vi "canDataSort.vi"() -> ()   [LabVIEW 2023] (continued)
  0CF103A7   00000004    8        17\t1F\t08\t60\tB1\t1F\t08\t66\r\n      4644  0C3C4D4A   00000004    8        BE\tFF\tFF\t7F\t18\tFF\tFF\t66\r\n      4643  0CF102A7   00000004    8        30\t75\tE0\t2E\t80\tFF\tFF\tFD\r\n      4642  0CF101A7   00000004    8        68\t00\t97\tCC\t00\t19\t39\t02\r\n      4649  18FEF117   00000004    8        F7\t97\tCC\tCF\tFF\tFF\tFF\tFF\r\n      4648  18FB01A7   00000004    8        FF\t1F\tFF\tFF\tFF\tFF\tFF\tFF\r\n      4648  18F121F0   00000004    8        09\t34\t00\t00\tFF\tFF\tB0\t01\r\n      4647  18F120F0   00000004    8        2B\t75\t60\tB1\tB0\t01\tFF\tFF\r\n      4646  18F108A7   00000004    8        F0\t00\t00\tFF\tFF\tFF\tFF\t47\r\n      4646  18F106A7   00000004    8        00\tF7\tFF\tFF\tFF\tFF\tFF\tCD\r\n      4645  0CF105A7   00000004    8        94\t11\t00\t55\tFF\tFF\tFF\t23\r\n      4645  0CF104A7   00000004    8        F0\t60\t22\tFC\tFF\tFF\tFF\t66\r\n      4644  0CF103A7   00000004    8        17\t1F\t08\t60\tB1\t1F\t08\t66\r\n      4644  0C3C4D4A   00000004    8        BE\tFF\tFF\t7F\t18\tFF\tFF\t66\r\n      4643  0CF102A7   00000004    8        30\t75\tE0\t2E\t80\tFF\tFF\tFD\r\n      4649  1FFFFFFF   00000004    8        00\t00\tFF\tFF\tFF\tFF\tFF\tFF\r\n      4649  18FEF117   00000004    8        F7\t97\tCC\tCF\tFF\tFF\tFF\tFF\r\n      4648  18FB01A7   00000004    8        FF\t1F\tFF\tFF\tFF\tFF\tFF\tFF\r\n      4648  18F121F0   00000004    8        09\t34\t00\t00\tFF\tFF\tB0\t01\r\n      4647  18F120F0   00000004    8        2B\t75\t60\tB1\tB0\t01\tFF\tFF\r\n      4646  18F108A7   00000004    8        F0\t00\t00\tFF\tFF\tFF\tFF\t47\r\n      4646  18F106A7   00000004    8        00\tF7\tFF\tFF\tFF\tFF\tFF\tCD\r\n      4645  0CF105A7   00000004    8        94\t11\t00\t55\tFF\tFF\tFF\t23\r\n      4645  0CF104A7   00000004    8        F0\t60\t22\tFC\tFF\tFF\tFF\t66\r\n      4644  0CF103A7   00000004    8        17\t1F\t08\t60\tB1\t1F\t08\t66\r\n      4644  0C3C4D4A   00000004    8        BE\tFF\tFF\t7F\t18\tFF\tFF\t66\r\n      4652  1FFFFFFF   00000004    8        00\t20\tFF\tFF\tFF\tFF\tFF\tFF\r\n      4649  1FFFFFFF   00000004    8        00\t00\tFF\tFF\tFF\tFF\tFF\tFF\r\n      4649  18FEF117   00000004    8        F7\t97\tCC\tCF\tFF\tFF\tFF\tFF\r\n      4648  18FB01A7   00000004    8        FF\t1F\tFF\tFF\tFF\tFF\tFF\tFF\r\n      4648  18F121F0   00000004    8        09\t34\t00\t00\tFF\tFF\tB0\t01\r\n      4647  18F120F0   00000004    8        2B\t75\t60\tB1\tB0\t01\tFF\tFF\r\n      4646  18F108A7   00000004    8        F0\t00\t00\tFF\tFF\tFF\tFF\t47\r\n      4646  18F106A7   00000004    8        00\tF7\tFF\tFF\tFF\tFF\tFF\tCD\r\n      4645  0CF105A7   00000004    8        94\t11\t00\t55\tFF\tFF\tFF\t23\r\n      4645  0CF104A7   00000004    8        F0\t60\t22\tFC\tFF\tFF\tFF\t66\r\n      4644  0CF103A7   00000004    8        17\t1F\t08\t60\tB1\t1F\t08\t66\r\n      4662  1FFFFFFF   00000004    8        00\t20\tFF\tFF\tFF\tFF\tFF\tFF\r\n      4652  1FFFFFFF   00000004    8        00\t20\tFF\tFF\tFF\tFF\tFF\tFF\r\n      4649  1FFFFFFF   00000004    8        00\t00\tFF\tFF\tFF\tFF\tFF\tFF\r\n      4649  18FEF117   00000004    8        F7\t97\tCC\tCF\tFF\tFF\tFF\tFF\r\n      4648  18FB01A7   00000004    8        FF\t1F\tFF\tFF\tFF\tFF\tFF\tFF\r\n      4648  18F121F0   00000004    8        09\t34\t00\t00\tFF\tFF\tB0\t01\r\n      4647  18F120F0   00000004    8        2B\t75\t60\tB1\tB0\t01\tFF\tFF\r\n      4646  18F108A7   00000004    8        F0\t00\t00\tFF\tFF\tFF\tFF\t47\r\n      4646  18F106A7   00000004    8        00\tF7\tFF\tFF\tFF\tFF\tFF\tCD\r\n      4645  0CF105A7   00000004    8        94\t11\t00\t55\tFF\tFF\tFF\t23\r\n      4645  0CF104A7   00000004    8        F0\t60\t22\tFC\tFF\tFF\tFF\t66\r\n      4662  0CF101A7   00000004    8        68\t00\t97\tCC\t00\t19\t39\t03\r\n      4662  1FFFFFFF   00000004    8        00\t20\tFF\tFF\tFF\tFF\tFF\tFF\r\n      4652  1FFFFFFF   00000004    8        00\t20\tFF\tFF\tFF\tFF\tFF\tFF\r\n      4649  1FFFFFFF   00000004    8        00\t00\tFF\tFF\tFF\tFF\tFF\tFF\r\n      4649  18FEF117   00000004    8        F7\t97\tCC\tCF\tFF\tFF\tFF\tFF\r\n      4648  18FB01A7   00000004    8        FF\t1F\tFF\tFF\tFF\tFF\tFF\tFF\r\n      4648  18F121F0   00000004    8        09\t34\t00\t00\tFF\tFF\tB0\t01\r\n      4647  18F120F0   00000004    8        2B\t75\t60\tB1\tB0\t01\tFF\tFF\r\n      4646  18F108A7   00000004    8        F0\t00\t00\tFF\tFF\tFF\tFF\t47\r\n      4646  18F106A7   00000004    8        00\tF7\tFF\tFF\tFF\tFF\tFF\tCD\r\n      4645  0CF105A7   00000004    8        94\t11\t00\t55\tFF\tFF\tFF\t23\r\n      4663  0CF102A7   00000004    8        30\t75\tE0\t2E\t80\tFF\tFF\tFD\r\n      4662  0CF101A7   00000004    8        68\t00\t97\tCC\t00\t19\t39\t03\r\n      4662  1FFFFFFF   00000004    8        00\t20\tFF\tFF\tFF\tFF\tFF\tFF\r\n      4652  1FFFFFFF   00000004    8        00\t20\tFF\tFF\tFF\tFF\tFF\tFF\r\n      4649  1FFFFFFF   00000004    8        00\t00\tFF\tFF\tFF\tFF\tFF\tFF\r\n      4649  18FEF117   00000004    8        F7\t97\tCC\tCF\tFF\tFF\tFF\tFF\r\n      4648  18FB01A7   00000004    8        FF\t1F\tFF\tFF\tFF\tFF\tFF\tFF\r\n      4648  18F121F0   00000004    8        09\t34\t00\t00\tFF\tFF\tB0\t01\r\n      4647  18F120F0   00000004    8        2B\t75\t60\tB1\tB0\t01\tFF\tFF\r\n      4646  18F108A7   00000004    8        F0\t00\t00\tFF\tFF\tFF\tFF\t47\r\n      4646  18F106A7   00000004    8        00\tF7\tFF\tFF\tFF\tFF\tFF\tCD\r\n      4672  1FFFFFFF   00000004    8        00\t20\tFF\tFF\tFF\tFF\tFF\tFF\r\n      4663  0CF102A7   00000004    8        30\t75\tE0\t2E\t80\tFF\tFF\tFD\r\n      4662  0CF101A7   00000004    8        68\t00\t97\tCC\t00\t19\t39\t03\r\n      4662  1FFFFFFF   00000004    8        00\t20\tFF\tFF\tFF\tFF\tFF\tFF\r\n      4652  1FFFFFFF   00000004    8        00\t20\tFF\tFF\tFF\tFF\tFF\tFF\r\n      4649  1FFFFFFF   00000004    8        00\t00\tFF\tFF\tFF\tFF\tFF\tFF\r\n      4649  18FEF117   00000004    8        F7\t97\tCC\tCF\tFF\tFF\tFF\tFF\r\n      4648  18FB01A7   00000004    8        FF\t1F\tFF\tFF\tFF\tFF\tFF\tFF\r\n      4648  18F121F0   00000004    8        09\t34\t00\t00\tFF\tFF\tB0\t01\r\n      4647  18F120F0   00000004    8        2B\t75\t60\tB1\tB0\t01\tFF\tFF\r\n      4646  18F108A7   00000004    8        F0\t00\t00\tFF\tFF\tFF\tFF\t47\r\n      4682  1FFFFFFF   00000004    8        00\t20\tFF\tFF\tFF\tFF\tFF\tFF\r\n      4672  1FFFFFFF   00000004    8        00\t20\tFF\tFF\tFF\tFF\tFF\tFF\r\n      4663  0CF102A7   00000004    8        30\t75\tE0\t2E\t80\tFF\tFF\tFD\r\n      4662  0CF101A7   00000004    8        68\t00\t97\tCC\t00\t19\t39\t03\r\n      4662  1FFFFFFF   00000004    8        00\t20\tFF\tFF\tFF\tFF\tFF\tFF\r\n      4652  1FFFFFFF   00000004    8        00\t20\tFF\tFF\tFF\tFF\tFF\tFF\r\n      4649  1FFFFFFF   00000004    8        00\t00\tFF\tFF\tFF\tFF\tFF\tFF\r\n      4649  18FEF117   00000004    8        F7\t97\tCC\tCF\tFF\tFF\tFF\tFF\r\n      4648  18FB01A7   00000004    8        FF\t1F\tFF\tFF\tFF\tFF\tFF\tFF\r\n      4648  18F121F0   00000004    8        09\t34\t00\t00\tFF\tFF\tB0\t01\r\n      4647  18F120F0   00000004    8        2B\t75\t60\tB1\tB0\t01\tFF\tFF\r\n      4683  0CF101A7   00000004    8        68\t00\t97\tCC\t00\t19\t39\t04\r\n      4682  1FFFFFFF   00000004    8        00\t20\tFF\tFF\tFF\tFF\tFF\tFF\r\n      4672  1FFFFFFF   00000004    8        00\t20\tFF\tFF\tFF\tFF\tFF\tFF\r\n      4663  0CF102A7   00000004    8        30\t75\tE0\t2E\t80\tFF\tFF\tFD\r\n      4662  0CF101A7   00000004    8        68\t00\t97\tCC\t00\t19\t39\t03\r\n      4662  1FFFFFFF   00000004    8        00\t20\tFF\tFF\tFF\tFF\tFF\tFF\r\n      4652  1FFFFFFF   00000004    8        00\t20\tFF\tFF\tFF\tFF\tFF\tFF\r\n      4649  1FFFFFFF   00000004    8        00\t00\tFF\tFF\tFF\tFF\tFF\tFF\r\n      4649  18FEF117   00000004    8        F7\t97\tCC\tCF\tFF\tFF\tFF\tFF\r\n      4648  18FB01A7   00000004    8        FF\t1F\tFF\tFF\tFF\tFF\tFF\tFF\r\n      4648  18F121F0   00000004    8        09\t34\t00\t00\tFF\tFF\tB0\t01\r\n      4683  0CF102A7   00000004    8        30\t75\tE0\t2E\t80\tFF\tFF\tFD\r\n      4683  0CF101A7   00000004    8        68\t00\t97\tCC\t00\t19\t39\t04\r\n      4682  1FFFFFFF   00000004    8        00\t20\tFF\tFF\tFF\tFF\tFF\tFF\r\n      4672  1FFFFFFF   00000004    8        00\t20\tFF\tFF\tFF\tFF\tFF\tFF\r\n      4663  0CF102A7   00000004    8        30\t75\tE0\t2E\t80\tFF\tFF\tFD\r\n      4662  0CF101A7   00000004    8        68\t00\t97\tCC\t00\t19\t39\t03\r\n      4662  1FFFFFFF   00000004    8        00\t20\tFF\tFF\tFF\tFF\tFF\tFF\r\n      4652  1FFFFFFF   00000004    8        00\t20\tFF\tFF\tFF\tFF\tFF\tFF\r\n      4649  1FFFFFFF   00000004    8        00\t00\tFF\tFF\tFF\tFF\tFF\tFF\r\n      4649  18FEF117   00000004    8        F7\t97\tCC\tCF\tFF\tFF\tFF\tFF\r\n      4648  18FB01A7   00000004    8        FF\t1F\tFF\tFF\tFF\tFF\tFF\tFF\r\n      4692  1FFFFFFF   00000004    8        00\t00\tFF\tFF\tFF\tFF\tFF\tFF\r\n      4683  0CF102A7   00000004    8        30\t75\tE0\t2E\t80\tFF\tFF\tFD\r\n      4683  0CF101A7   00000004    8        68\t00\t97\tCC\t00\t19\t39\t04\r\n      4682  1FFFFFFF   00000004    8        00\t20\tFF\tFF\tFF\tFF\tFF\tFF\r\n      4672  1FFFFFFF   00000004    8        00\t20\tFF\tFF\tFF\tFF\tFF\tFF\r\n      4663  0CF102A7   00000004    8        30\t75\tE0\t2E\t80\tFF\tFF\tFD\r\n      4662  0CF101A7   00000004    8        68\t00\t97\tCC\t00\t19\t39\t03\r\n      4662  1FFFFFFF   00000004    8        00\t20\tFF\tFF\tFF\tFF\tFF\tFF\r\n      4652  1FFFFFFF   00000004    8        00\t20\tFF\tFF\tFF\tFF\tFF\tFF\r\n      4649  1FFFFFFF   00000004    8        00\t00\tFF\tFF\tFF\tFF\tFF\tFF\r\n      4649  18FEF117   00000004    8        F7\t97\tCC\tCF\tFF\tFF\tFF\tFF\r\n      4693  18F106A7   00000004    8        00\tF7\tFF\tFF\tFF\tFF\tFF\tCE\r\n      4692  1FFFFFFF   00000004    8        00\t00\tFF\tFF\tFF\tFF\tFF\tFF\r\n      4683  0CF102A7   00000004    8        30\t75\tE0\t2E\t80\tFF\tFF\tFD\r\n      4683  0CF101A7   00000004    8        68\t00\t97\tCC\t00\t19\t39\t04\r\n      4682  1FFFFFFF   00000004    8        00\t20\tFF\tFF\tFF\tFF\tFF\tFF\r\n      4672  1FFFFFFF   00000004    8        00\t20\tFF\tFF\tFF\tFF\tFF\tFF\r\n      4663  0CF102A7   00000004    8        30\t75\tE0\t2E\t80\tFF\tFF\tFD\r\n      4662  0CF101A7   00000004    8        68\t00\t97\tCC\t00\t19\t39\t03\r\n      4662  1FFFFFFF   00000004    8        00\t20\tFF\tFF\tFF\tFF\tFF\tFF\r\n      4652  1FFFFFFF   00000004    8        00\t20\tFF\tFF\tFF\tFF\tFF\tFF\r\n      4649  1FFFFFFF   00000004    8        00\t00\tFF\tFF\tFF\tFF\tFF\tFF\r\n      4702  1FFFFFFF   00000004    8        00\t20\tFF\tFF\tFF\tFF\tFF\tFF\r\n      4693  18F106A7   00000004    8        00\tF7\tFF\tFF\tFF\tFF\tFF\tCE\r\n      4692  1FFFFFFF   00000004    8        00\t00\tFF\tFF\tFF\tFF\tFF\tFF\r\n      4683  0CF102A7   00000004    8        30\t75\tE0\t2E\t80\tFF\tFF\tFD\r\n      4683  0CF101A7   00000004    8        68\t00\t97\tCC\t00\t19\t39\t04\r\n      4682  1FFFFFFF   00000004    8        00\t20\tFF\tFF\tFF\tFF\tFF\tFF\r\n      4672  1FFFFFFF   00000004    8        00\t20\tFF\tFF\tFF\tFF\tFF\tFF\r\n      4663  0CF102A7   00000004    8        30\t75\tE0\t2E\t80\tFF\tFF\tFD\r\n      4662  0CF101A7   00000004    8        68\t00\t97\tCC\t00\t19\t39\t03\r\n      4662  1FFFFFFF   00000004    8        00\t20\tFF\tFF\tFF\tFF\tFF\tFF\r\n      4652  1FFFFFFF   00000004    8        00\t20\tFF\tFF\tFF\tFF\tFF\tFF\r\n      4702  0CF101A7   00000004    8        68\t00\t97\tCC\t00\t19\t39\t05\r\n      4702  1FFFFFFF   00000004    8        00\t20\tFF\tFF\tFF\tFF\tFF\tFF\r\n      4693  18F106A7   00000004    8        00\tF7\tFF\tFF\tFF\tFF\tFF\tCE\r\n      4692  1FFFFFFF   00000004    8        00\t00\tFF\tFF\tFF\tFF\tFF\tFF\r\n      4683  0CF102A7   00000004    8        30\t75\tE0\t2E\t80\tFF\tFF\tFD\r\n      4683  0CF101A7   00000004    8        68\t00\t97\tCC\t00\t19\t39\t04\r\n      4682  1FFFFFFF   00000004    8        00\t20\tFF\tFF\tFF\tFF\tFF\tFF\r\n      4672  1FFFFFFF   00000004    8        00\t20\tFF\tFF\tFF\tFF\tFF\tFF\r\n      4663  0CF102A7   00000004    8        30\t75\tE0\t2E\t80\tFF\tFF\tFD\r\n      4662  0CF101A7   00000004    8        68\t00\t97\tCC\t00\t19\t39\t03\r\n      4662  1FFFFFFF   00000004    8        00\t20\tFF\tFF\tFF\tFF\tFF\tFF\r\n" caption="String"
  in  "Array":T1(array[cluster])=[{"1429FF9B", "Frame"="AirCompr1\ndatabase", "NameShort"="AirCompr1Curr", "StartBit"=32, "NumBits"=8, "Min"=0.0, "Max"=100.0, "ScaleFac"=1.0, "ScaleOff"=0.0}, {"1429FF9B", "Frame"="AirCompr1\ndatabase", "NameShort"="AirCompr1ErrCode", "StartBit"=56, "NumBits"=4, "Min"=0.0, "Max"=1.0, "ScaleFac"=1.0, "ScaleOff"=0.0}, {"1429FF9B", "Frame"="AirCompr1\ndatabase", "NameShort"="AirCompr1Life", "StartBit"=48, "NumBits"=8, "Min"=0.0, "Max"=255.0, "ScaleFac"=1.0, "ScaleOff"=0.0}, {"1429FF9B", "Frame"="AirCompr1\ndatabase", "NameShort"="AirCompr1MtrSpeed", "StartBit"=0, "NumBits"=16, "Min"=0.0, "Max"=5000.0, "ScaleFac"=0.125, "ScaleOff"=0.0}, {"1429FF9B", "Frame"="AirCompr1\ndatabase", "NameShort"="AirCompr1PrechgStat", "StartBit"=63, "NumBits"=1, "Min"=0.0, "Max"=1.0, "ScaleFac"=1.0, "ScaleOff"=0.0}, {"1429FF9B", "Frame"="AirCompr1\ndatabase", "NameShort"="AirCompr1Stat", "StartBit"=60, "NumBits"=2, "Min"=0.0, "Max"=1.0, "ScaleFac"=1.0, "ScaleOff"=0.0}, {"1429FF9B", "Frame"="AirCompr1\ndatabase", "NameShort"="AirCompr1Temp", "StartBit"=40, "NumBits"=8, "Min"=-40.0, "Max"=210.0, "ScaleFac"=1.0, "ScaleOff"=-40.0}, {"1429FF9B", "Frame"="AirCompr1\ndatabase", "NameShort"="AirCompr1Volt", "StartBit"=16, "NumBits"=16, "Min"=0.0, "Max"=1000.0, "ScaleFac"=0.1, "ScaleOff"=0.0}, {"18FFC09E", "Frame"="AirCon\ndatabase", "NameShort"="AirConCommWarn", "StartBit"=47, "NumBits"=1, "Min"=0.0, "Max"=1.0, "ScaleFac"=1.0, "ScaleOff"=0.0}, {"18FFC09E", "Frame"="AirCon\ndatabase", "NameShort"="AirConCooling1DefrostValidation", "StartBit"=17, "NumBits"=1, "Min"=0.0, "Max"=1.0, "ScaleFac"=1.0, "ScaleOff"=0.0}, {"18FFC09E", "Frame"="AirCon\ndatabase", "NameShort"="AirConCooling1Validation", "StartBit"=23, "NumBits"=1, "Min"=0.0, "Max"=1.0, "ScaleFac"=1.0, "ScaleOff"=0.0}, {"18FFC09E", "Frame"="AirCon\ndatabase", "NameShort"="AirConCooling2DefrostValidation", "StartBit"=20, "NumBits"=1, "Min"=0.0, "Max"=1.0, "ScaleFac"=1.0, "ScaleOff"=0.0}, {"18FFC09E", "Frame"="AirCon\ndatabase", "NameShort"="AirConCooling2Validation", "StartBit"=21, "NumBits"=1, "Min"=0.0, "Max"=1.0, "ScaleFac"=1.0, "ScaleOff"=0.0}, {"18FFC09E", "Frame"="AirCon\ndatabase", "NameShort"="AirConEvaporator1SnsrOpenCircuit", "StartBit"=2, "NumBits"=1, "Min"=0.0, "Max"=1.0, "ScaleFac"=1.0, "ScaleOff"=0.0}, {"18FFC09E", "Frame"="AirCon\ndatabase", "NameShort"="AirConEvaporator2SnsrOpenCircuit", "StartBit"=3, "NumBits"=1, "Min"=0.0, "Max"=1.0, "ScaleFac"=1.0, "ScaleOff"=0.0}, {"18FFC09E", "Frame"="AirCon\ndatabase", "NameShort"="AirConHeatValidation", "StartBit"=16, "NumBits"=1, "Min"=0.0, "Max"=1.0, "ScaleFac"=1.0, "ScaleOff"=0.0}, {"18FFC09E", "Frame"="AirCon\ndatabase", "NameShort"="AirConHighSpeed", "StartBit"=15, "NumBits"=1, "Min"=0.0, "Max"=1.0, "ScaleFac"=1.0, "ScaleOff"=0.0}, {"18FFC09E", "Frame"="AirCon\ndatabase", "NameShort"="AirConIndoorTemp", "StartBit"=24, "NumBits"=8, "Min"=-30.0, "Max"=97.0, "ScaleFac"=0.5, "ScaleOff"=-30.0}, {"18FFC09E", "Frame"="AirCon\ndatabase", "NameShort"="AirConInverterFailure", "StartBit"=6, "NumBits"=1, "Min"=0.0, "Max"=1.0, "ScaleFac"=1.0, "ScaleOff"=0.0}, {"18FFC09E", "Frame"="AirCon\ndatabase", "NameShort"="AirConLife", "StartBit"=56, "NumBits"=8, "Min"=0.0, "Max"=255.0, "ScaleFac"=1.0, "ScaleOff"=0.0}, {"18FFC09E", "Frame"="AirCon\ndatabase", "NameShort"="AirConLowSpeed", "StartBit"=13, "NumBits"=1, "Min"=0.0, "Max"=1.0, "ScaleFac"=1.0, "ScaleOff"=0.0}, {"18FFC09E", "Frame"="AirCon\ndatabase", "NameShort"="AirConMidSpeed", "StartBit"=14, "NumBits"=1, "Min"=0.0, "Max"=1.0, "ScaleFac"=1.0, "ScaleOff"=0.0}, {"18FFC09E", "Frame"="AirCon\ndatabase", "NameShort"="AirConOutTempSensorOpenCircuit", "StartBit"=1, "NumBits"=1, "Min"=0.0, "Max"=1.0, "ScaleFac"=1.0, "ScaleOff"=0.0}, {"18FFC09E", "Frame"="AirCon\ndatabase", "NameShort"="AirConOutdoorTemp", "StartBit"=32, "NumBits"=8, "Min"=-30.0, "Max"=97.0, "ScaleFac"=0.5, "ScaleOff"=-30.0}, {"18FFC09E", "Frame"="AirCon\ndatabase", "NameShort"="AirConPowSupplyOverVolt", "StartBit"=4, "NumBits"=1, "Min"=0.0, "Max"=1.0, "ScaleFac"=1.0, "ScaleOff"=0.0}, {"18FFC09E", "Frame"="AirCon\ndatabase", "NameShort"="AirConPowSupplyUnderVolt", "StartBit"=5, "NumBits"=1, "Min"=0.0, "Max"=1.0, "ScaleFac"=1.0, "ScaleOff"=0.0}, {"18FFC09E", "Frame"="AirCon\ndatabase", "NameShort"="AirConPressureFailure", "StartBit"=7, "NumBits"=1, "Min"=0.0, "Max"=1.0, "ScaleFac"=1.0, "ScaleOff"=0.0}, {"18FFC09E", "Frame"="AirCon\ndatabase", "NameShort"="AirConReqHV", "StartBit"=55, "NumBits"=1, "Min"=0.0, "Max"=1.0, "ScaleFac"=1.0, "ScaleOff"=0.0}, {"18FFC09E", "Frame"="AirCon\ndatabase", "NameShort"="AirConSterilizationValidation", "StartBit"=19, "NumBits"=1, "Min"=0.0, "Max"=1.0, "ScaleFac"=1.0, "ScaleOff"=0.0}, {"18FFC09E", "Frame"="AirCon\ndatabase", "NameShort"="AirConTempSensorOpenCircuit", "StartBit"=0, "NumBits"=1, "Min"=0.0, "Max"=1.0, "ScaleFac"=1.0, "ScaleOff"=0.0}, {"18FFC09E", "Frame"="AirCon\ndatabase", "NameShort"="AirConVentilatorValidation", "StartBit"=18, "NumBits"=1, "Min"=0.0, "Max"=1.0, "ScaleFac"=1.0, "ScaleOff"=0.0}, {"CFFE2A0", "Frame"="BCMData1\ndatabase", "NameShort"="BCMBatteryCoolantTemperature", "StartBit"=16, "NumBits"=8, "Min"=-40.0, "Max"=210.0, "ScaleFac"=1.0, "ScaleOff"=-40.0}, {"CFFE2A0", "Frame"="BCMData1\ndatabase", "NameShort"="BCMFrontAirReservoirPressure", "StartBit"=24, "NumBits"=8, "Min"=0.0, "Max"=2000.0, "ScaleFac"=8.0, "ScaleOff"=0.0}, {"CFFE2A0", "Frame"="BCMData1\ndatabase", "NameShort"="BCMLeadAcidBatteryVoltage", "StartBit"=0, "NumBits"=8, "Min"=0.0, "Max"=50.0, "ScaleFac"=0.2, "ScaleOff"=0.0}, {"CFFE2A0", "Frame"="BCMData1\ndatabase", "NameShort"="BCMMotorCoolantTemperature", "StartBit"=8, "NumBits"=8, "Min"=-40.0, "Max"=210.0, "ScaleFac"=1.0, "ScaleOff"=-40.0}, {"CFFE2A0", "Frame"="BCMData1\ndatabase", "NameShort"="BCMRearAirReservoirPressure", "StartBit"=32, "NumBits"=8, "Min"=0.0, "Max"=2000.0, "ScaleFac"=8.0, "ScaleOff"=0.0}, {"CFFE1A0", "Frame"="BCMIO1\ndatabase", "NameShort"="BCMABSActuation", "StartBit"=50, "NumBits"=2, "Min"=0.0, "Max"=3.0, "ScaleFac"=1.0, "ScaleOff"=0.0}, {"CFFE1A0", "Frame"="BCMIO1\ndatabase", "NameShort"="BCMAlcoholInterlock", "StartBit"=48, "NumBits"=2, "Min"=0.0, "Max"=3.0, "ScaleFac"=1.0, "ScaleOff"=0.0}, {"CFFE1A0", "Frame"="BCMIO1\ndatabase", "NameShort"="BCMAutoHeadLight", "StartBit"=60, "NumBits"=2, "Min"=0.0, "Max"=3.0, "ScaleFac"=1.0, "ScaleOff"=0.0}, {"CFFE1A0", "Frame"="BCMIO1\ndatabase", "NameShort"="BCMBrakePadWarning", "StartBit"=52, "NumBits"=2, "Min"=0.0, "Max"=3.0, "ScaleFac"=1.0, "ScaleOff"=0.0}, {"CFFE1A0", "Frame"="BCMIO1\ndatabase", "NameShort"="BCMBrakeRegeneration", "StartBit"=32, "NumBits"=2, "Min"=0.0, "Max"=3.0, "ScaleFac"=1.0, "ScaleOff"=0.0}, {"CFFE1A0", "Frame"="BCMIO1\ndatabase", "NameShort"="BCMCallHelp", "StartBit"=16, "NumBits"=2, "Min"=0.0, "Max"=3.0, "ScaleFac"=1.0, "ScaleOff"=0.0}, {"CFFE1A0", "Frame"="BCMIO1\ndatabase", "NameShort"="BCMDoorSwitchCoverEmergency", "StartBit"=26, "NumBits"=2, "Min"=0.0, "Max"=3.0, "ScaleFac"=1.0, "ScaleOff"=0.0}, {"CFFE1A0", "Frame"="BCMIO1\ndatabase", "NameShort"="BCMECASKneeling", "StartBit"=36, "NumBits"=2, "Min"=0.0, "Max"=3.0, "ScaleFac"=1.0, "ScaleOff"=0.0}, {"CFFE1A0", "Frame"="BCMIO1\ndatabase", "NameShort"="BCMECASWarning", "StartBit"=38, "NumBits"=2, "Min"=0.0, "Max"=3.0, "ScaleFac"=1.0, "ScaleOff"=0.0}, {"CFFE1A0", "Frame"="BCMIO1\ndatabase", "NameShort"="BCMEmergencyStop", "StartBit"=44, "NumBits"=2, "Min"=0.0, "Max"=3.0, "ScaleFac"=1.0, "ScaleOff"=0.0}, {"CFFE1A0", "Frame"="BCMIO1\ndatabase", "NameShort"="BCMEscapeDoorOpen", "StartBit"=56, "NumBits"=2, "Min"=0.0, "Max"=3.0, "ScaleFac"=1.0, "ScaleOff"=0.0}, {"CFFE1A0", "Frame"="BCMIO1\ndatabase", "NameShort"="BCMFootBrake", "StartBit"=54, "NumBits"=2, "Min"=0.0, "Max"=3.0, "ScaleFac"=1.0, "ScaleOff"=0.0}, {"CFFE1A0", "Frame"="BCMIO1\ndatabase", "NameShort"="BCMFrontDoor", "StartBit"=18, "NumBits"=2, "Min"=0.0, "Max"=3.0, "ScaleFac"=1.0, "ScaleOff"=0.0}, {"CFFE1A0", "Frame"="BCMIO1\ndatabase", "NameShort"="BCMFrontDoorEmergencyOpen", "StartBit"=22, "NumBits"=2, "Min"=0.0, "Max"=3.0, "ScaleFac"=1.0, "ScaleOff"=0.0}, {"CFFE1A0", "Frame"="BCMIO1\ndatabase", "NameShort"="BCMFrontFogLight", "StartBit"=12, "NumBits"=2, "Min"=0.0, "Max"=3.0, "ScaleFac"=1.0, "ScaleOff"=0.0}, {"CFFE1A0", "Frame"="BCMIO1\ndatabase", "NameShort"="BCMFrontWindowDefog", "StartBit"=28, "NumBits"=2, "Min"=0.0, "Max"=3.0, "ScaleFac"=1.0, "ScaleOff"=0.0}, {"CFFE1A0", "Frame"="BCMIO1\ndatabase", "NameShort"="BCMHandBrake", "StartBit"=34, "NumBits"=2, "Min"=0.0, "Max"=3.0, "ScaleFac"=1.0, "ScaleOff"=0.0}, {"CFFE1A0", "Frame"="BCMIO1\ndatabase", "NameShort"="BCMHazardLight", "StartBit"=10, "NumBits"=2, "Min"=0.0, "Max"=3.0, "ScaleFac"=1.0, "ScaleOff"=0.0}, {"CFFE1A0", "Frame"="BCMIO1\ndatabase", "NameShort"="BCMHighBeams", "StartBit"=6, "NumBits"=2, "Min"=0.0, "Max"=3.0, "ScaleFac"=1.0, "ScaleOff"=0.0}, {"CFFE1A0", "Frame"="BCMIO1\ndatabase", "NameShort"="BCMLowBeams", "StartBit"=4, "NumBits"=2, "Min"=0.0, "Max"=3.0, "ScaleFac"=1.0, "ScaleOff"=0.0}, {"CFFE1A0", "Frame"="BCMIO1\ndatabase", "NameShort"="BCMMiddleDoor", "StartBit"=20, "NumBits"=2, "Min"=0.0, "Max"=3.0, "ScaleFac"=1.0, "ScaleOff"=0.0}, {"CFFE1A0", "Frame"="BCMIO1\ndatabase", "NameShort"="BCMMiddleDoorEmergencyOpen", "StartBit"=24, "NumBits"=2, "Min"=0.0, "Max"=3.0, "ScaleFac"=1.0, "ScaleOff"=0.0}, {"CFFE1A0", "Frame"="BCMIO1\ndatabase", "NameShort"="BCMMirrorDefog", "StartBit"=30, "NumBits"=2, "Min"=0.0, "Max"=3.0, "ScaleFac"=1.0, "ScaleOff"=0.0}, {"CFFE1A0", "Frame"="BCMIO1\ndatabase", "NameShort"="BCMPositionLight", "StartBit"=8, "NumBits"=2, "Min"=0.0, "Max"=3.0, "ScaleFac"=1.0, "ScaleOff"=0.0}, {"CFFE1A0", "Frame"="BCMIO1\ndatabase", "NameShort"="BCMRampBoard", "StartBit"=46, "NumBits"=2, "Min"=0.0, "Max"=3.0, "ScaleFac"=1.0, "ScaleOff"=0.0}, {"CFFE1A0", "Frame"="BCMIO1\ndatabase", "NameShort"="BCMRearFogLight", "StartBit"=14, "NumBits"=2, "Min"=0.0, "Max"=3.0, "ScaleFac"=1.0, "ScaleOff"=0.0}, {"CFFE1A0", "Frame"="BCMIO1\ndatabase", "NameShort"="BCMRearHatchOpen", "StartBit"=42, "NumBits"=2, "Min"=0.0, "Max"=3.0, "ScaleFac"=1.0, "ScaleOff"=0.0}, {"CFFE1A0", "Frame"="BCMIO1\ndatabase", "NameShort"="BCMReversingLight", "StartBit"=62, "NumBits"=2, "Min"=0.0, "Max"=3.0, "ScaleFac"=1.0, "ScaleOff"=0.0}, {"CFFE1A0", "Frame"="BCMIO1\ndatabase", "NameShort"="BCMRunningLight", "StartBit"=58, "NumBits"=2, "Min"=0.0, "Max"=3.0, "ScaleFac"=1.0, "ScaleOff"=0.0}, {"CFFE1A0", "Frame"="BCMIO1\ndatabase", "NameShort"="BCMStopBell", "StartBit"=40, "NumBits"=2, "Min"=0.0, "Max"=3.0, "ScaleFac"=1.0, "ScaleOff"=0.0}, {"CFFE1A0", "Frame"="BCMIO1\ndatabase", "NameShort"="BCMTurnLeft", "StartBit"=0, "NumBits"=2, "Min"=0.0, "Max"=3.0, "ScaleFac"=1.0, "ScaleOff"=0.0}, {"CFFE1A0", "Frame"="BCMIO1\ndatabase", "NameShort"="BCMTurnRight", "StartBit"=2, "NumBits"=2, "Min"=0.0, "Max"=3.0, "ScaleFac"=1.0, "ScaleOff"=0.0}, {"CFFD1A0", "Frame"="BCMIO2\ndatabase", "NameShort"="BCMKeySwitchACC", "StartBit"=2, "NumBits"=2, "Min"=0.0, "Max"=3.0, "ScaleFac"=1.0, "ScaleOff"=0.0}, {"CFFD1A0", "Frame"="BCMIO2\ndatabase", "NameShort"="BCMKeySwitchON", "StartBit"=4, "NumBits"=2, "Min"=0.0, "Max"=3.0, "ScaleFac"=1.0, "ScaleOff"=0.0}, {"CFFD1A0", "Frame"="BCMIO2\ndatabase", "NameShort"="BCMRoofEscapeWindowOpen", "StartBit"=8, "NumBits"=2, "Min"=0.0, "Max"=3.0, "ScaleFac"=1.0, "ScaleOff"=0.0}, {"CFFD1A0", "Frame"="BCMIO2\ndatabase", "NameShort"="BCMSeatBelt", "StartBit"=0, "NumBits"=2, "Min"=0.0, "Max"=3.0, "ScaleFac"=1.0, "ScaleOff"=0.0}, {"CFFD1A0", "Frame"="BCMIO2\ndatabase", "NameShort"="BCMSideEscapeWindowOpen", "StartBit"=10, "NumBits"=2, "Min"=0.0, "Max"=3.0, "ScaleFac"=1.0, "ScaleOff"=0.0}, {"CFFD1A0", "Frame"="BCMIO2\ndatabase", "NameShort"="BCMSteerWheelDetect", "StartBit"=6, "NumBits"=2, "Min"=0.0, "Max"=3.0, "ScaleFac"=1.0, "ScaleOff"=0.0}, {"18F13DF3", "Frame"="BMS01StatNRelay\ndatabase", "NameShort"="BMS01AirComprNDCDCNEhpsRelayStat", "StartBit"=59, "NumBits"=1, "Min"=0.0, "Max"=1.0, "ScaleFac"=1.0, "ScaleOff"=0.0}, {"18F13DF3", "Frame"="BMS01StatNRelay\ndatabase", "NameShort"="BMS01AirConRelayStat", "StartBit"=60, "NumBits"=1, "Min"=0.0, "Max"=1.0, "ScaleFac"=1.0, "ScaleOff"=0.0}, {"18F13DF3", "Frame"="BMS01StatNRelay\ndatabase", "NameShort"="BMS01BMSErrLv", "StartBit"=48, "NumBits"=3, "Min"=0.0, "Max"=1.0, "ScaleFac"=1.0, "ScaleOff"=0.0}, {"18F13DF3", "Frame"="BMS01StatNRelay\ndatabase", "NameShort"="BMS01BMSHVEmergCutoff", "StartBit"=56, "NumBits"=1, "Min"=0.0, "Max"=1.0, "ScaleFac"=1.0, "ScaleOff"=0.0}, {"18F13DF3", "Frame"="BMS01StatNRelay\ndatabase", "NameShort"="BMS01BMSPowerOffRequest", "StartBit"=51, "NumBits"=2, "Min"=0.0, "Max"=3.0, "ScaleFac"=1.0, "ScaleOff"=0.0}, {"18F13DF3", "Frame"="BMS01StatNRelay\ndatabase", "NameShort"="BMS01BMSSOC", "StartBit"=32, "NumBits"=16, "Min"=0.0, "Max"=100.0, "ScaleFac"=0.4, "ScaleOff"=0.0}, {"18F13DF3", "Frame"="BMS01StatNRelay\ndatabase", "NameShort"="BMS01BMSStat", "StartBit"=53, "NumBits"=3, "Min"=0.0, "Max"=7.0, "ScaleFac"=1.0, "ScaleOff"=0.0}, {"18F13DF3", "Frame"="BMS01StatNRelay\ndatabase", "NameShort"="BMS01BattChgRelayStat", "StartBit"=62, "NumBits"=1, "Min"=0.0, "Max"=1.0, "ScaleFac"=1.0, "ScaleOff"=0.0}, {"18F13DF3", "Frame"="BMS01StatNRelay\ndatabase", "NameShort"="BMS01BattCurr", "StartBit"=16, "NumBits"=16, "Min"=-1000.0, "Max"=1000.0, "ScaleFac"=0.1, "ScaleOff"=-1000.0}, {"18F13DF3", "Frame"="BMS01StatNRelay\ndatabase", "NameShort"="BMS01BattMainRelayStat", "StartBit"=63, "NumBits"=1, "Min"=0.0, "Max"=1.0, "ScaleFac"=1.0, "ScaleOff"=0.0}, {"18F13DF3", "Frame"="BMS01StatNRelay\ndatabase", "NameShort"="BMS01BattVolt", "StartBit"=0, "NumBits"=16, "Min"=0.0, "Max"=1000.0, "ScaleFac"=0.1, "ScaleOff"=0.0}, {"18F13DF3", "Frame"="BMS01StatNRelay\ndatabase", "NameShort"="BMS01DefrostRelayStat", "StartBit"=61, "NumBits"=1, "Min"=0.0, "Max"=1.0, "ScaleFac"=1.0, "ScaleOff"=0.0}, {"18F13DF3", "Frame"="BMS01StatNRelay\ndatabase", "NameShort"="BMS01MtrRelayStat", "StartBit"=58, "NumBits"=1, "Min"=0.0, "Max"=1.0, "ScaleFac"=1.0, "ScaleOff"=0.0}, {"18F13DF3", "Frame"="BMS01StatNRelay\ndatabase", "NameShort"="BMS01PrechgRelayStat", "StartBit"=57, "NumBits"=1, "Min"=0.0, "Max"=1.0, "ScaleFac"=1.0, "ScaleOff"=0.0}, {"18F13EF3", "Frame"="BMS02VoltDiff\ndatabase", "NameShort"="BMS02BattCellMaxTemp", "StartBit"=32, "NumBits"=8, "Min"=-40.0, "Max"=210.0, "ScaleFac"=1.0, "ScaleOff"=-40.0}, {"18F13EF3", "Frame"="BMS02VoltDiff\ndatabase", "NameShort"="BMS02BattCellMaxVolt", "StartBit"=0, "NumBits"=16, "Min"=0.0, "Max"=655.35, "ScaleFac"=0.01, "ScaleOff"=0.0}, {"18F13EF3", "Frame"="BMS02VoltDiff\ndatabase", "NameShort"="BMS02BattCellMinTemp", "StartBit"=40, "NumBits"=8, "Min"=-40.0, "Max"=210.0, "ScaleFac"=1.0, "ScaleOff"=-40.0}, {"18F13EF3", "Frame"="BMS02VoltDiff\ndatabase", "NameShort"="BMS02BattCellMinVolt", "StartBit"=16, "NumBits"=16, "Min"=0.0, "Max"=655.35, "ScaleFac"=0.01, "ScaleOff"=0.0}, {"18F13EF3", "Frame"="BMS02VoltDiff\ndatabase", "NameShort"="BMS02BattNominalCapacitykWh", "StartBit"=48, "NumBits"=16, "Min"=0.0, "Max"=65535.0, "ScaleFac"=1.0, "ScaleOff"=0.0}, {"18F140F3", "Frame"="BMS04Curr\ndatabase", "NameShort"="BMS04BattMaxChgCurr", "StartBit"=0, "NumBits"=16, "Min"=-1000.0, "Max"=1000.0, "ScaleFac"=0.1, "ScaleOff"=-1000.0}, {"18F140F3", "Frame"="BMS04Curr\ndatabase", "NameShort"="BMS04BattMaxDischgCurr", "StartBit"=16, "NumBits"=16, "Min"=-1000.0, "Max"=1000.0, "ScaleFac"=0.1, "ScaleOff"=-1000.0}, {"18F140F3", "Frame"="BMS04Curr\ndatabase", "NameShort"="BMS04BattMinSOCAllowed", "StartBit"=48, "NumBits"=8, "Min"=0.0, "Max"=100.0, "ScaleFac"=0.4, "ScaleOff"=0.0}, {"18F140F3", "Frame"="BMS04Curr\ndatabase", "NameShort"="BMS04BattPackAllowedMaxTemp", "StartBit"=32, "NumBits"=8, "Min"=-40.0, "Max"=210.0, "ScaleFac"=1.0, "ScaleOff"=-40.0}, {"18F140F3", "Frame"="BMS04Curr\ndatabase", "NameShort"="BMS04BattPackAllowedMinTemp", "StartBit"=40, "NumBits"=8, "Min"=-40.0, "Max"=210.0, "ScaleFac"=1.0, "ScaleOff"=-40.0}, {"18F141F3", "Frame"="BMS05Error\ndatabase", "NameShort"="BMS05BalanceSysStat", "StartBit"=24, "NumBits"=1, "Min"=0.0, "Max"=1.0, "ScaleFac"=1.0, "ScaleOff"=0.0}, {"18F141F3", "Frame"="BMS05Error\ndatabase", "NameShort"="BMS05BattCellOvervoltWarn", "StartBit"=12, "NumBits"=1, "Min"=0.0, "Max"=1.0, "ScaleFac"=1.0, "ScaleOff"=0.0}, {"18F141F3", "Frame"="BMS05Error\ndatabase", "NameShort"="BMS05BattCellUndervoltWarn", "StartBit"=13, "NumBits"=1, "Min"=0.0, "Max"=1.0, "ScaleFac"=1.0, "ScaleOff"=0.0}, {"18F141F3", "Frame"="BMS05Error\ndatabase", "NameShort"="BMS05BattCellVoltDiffWarn", "StartBit"=14, "NumBits"=1, "Min"=0.0, "Max"=1.0, "ScaleFac"=1.0, "ScaleOff"=0.0}, {"18F141F3", "Frame"="BMS05Error\ndatabase", "NameShort"="BMS05BowTypeChgStat", "StartBit"=40, "NumBits"=3, "Min"=0.0, "Max"=1.0, "ScaleFac"=1.0, "ScaleOff"=0.0}, {"18F141F3", "Frame"="BMS05Error\ndatabase", "NameShort"="BMS05CANVer", "StartBit"=56, "NumBits"=8, "Min"=0.0, "Max"=2.55, "ScaleFac"=0.01, "ScaleOff"=0.0}, {"18F141F3", "Frame"="BMS05Error\ndatabase", "NameShort"="BMS05ChgStat", "StartBit"=25, "NumBits"=2, "Min"=0.0, "Max"=1.0, "ScaleFac"=1.0, "ScaleOff"=0.0}, {"18F141F3", "Frame"="BMS05Error\ndatabase", "NameShort"="BMS05ChgSysMismatchWarn", "StartBit"=20, "NumBits"=1, "Min"=0.0, "Max"=1.0, "ScaleFac"=1.0, "ScaleOff"=0.0}, {"18F141F3", "Frame"="BMS05Error\ndatabase", "NameShort"="BMS05ErrCode", "StartBit"=0, "NumBits"=8, "Min"=0.0, "Max"=255.0, "ScaleFac"=1.0, "ScaleOff"=0.0}, {"18F141F3", "Frame"="BMS05Error\ndatabase", "NameShort"="BMS05HVInterlockDisconnectWarn", "StartBit"=21, "NumBits"=1, "Min"=0.0, "Max"=1.0, "ScaleFac"=1.0, "ScaleOff"=0.0}, {"18F141F3", "Frame"="BMS05Error\ndatabase", "NameShort"="BMS05HighTempWarn", "StartBit"=9, "NumBits"=1, "Min"=0.0, "Max"=1.0, "ScaleFac"=1.0, "ScaleOff"=0.0}, {"18F141F3", "Frame"="BMS05Error\ndatabase", "NameShort"="BMS05InsulationWarn", "StartBit"=19, "NumBits"=1, "Min"=0.0, "Max"=1.0, "ScaleFac"=1.0, "ScaleOff"=0.0}, {"18F141F3", "Frame"="BMS05Error\ndatabase", "NameShort"="BMS05Life", "StartBit"=48, "NumBits"=8, "Min"=0.0, "Max"=255.0, "ScaleFac"=1.0, "ScaleOff"=0.0}, {"18F141F3", "Frame"="BMS05Error\ndatabase", "NameShort"="BMS05OverChgWarn", "StartBit"=15, "NumBits"=1, "Min"=0.0, "Max"=1.0, "ScaleFac"=1.0, "ScaleOff"=0.0}, {"18F141F3", "Frame"="BMS05Error\ndatabase", "NameShort"="BMS05OvervoltWarn", "StartBit"=10, "NumBits"=1, "Min"=0.0, "Max"=1.0, "ScaleFac"=1.0, "ScaleOff"=0.0}, {"18F141F3", "Frame"="BMS05Error\ndatabase", "NameShort"="BMS05PluginStat", "StartBit"=32, "NumBits"=8, "Min"=0.0, "Max"=255.0, "ScaleFac"=1.0, "ScaleOff"=0.0}, {"18F141F3", "Frame"="BMS05Error\ndatabase", "NameShort"="BMS05SOCRadicalChangeWarn", "StartBit"=18, "NumBits"=1, "Min"=0.0, "Max"=1.0, "ScaleFac"=1.0, "ScaleOff"=0.0}, {"18F141F3", "Frame"="BMS05Error\ndatabase", "NameShort"="BMS05SOCTooHighWarn", "StartBit"=17, "NumBits"=1, "Min"=0.0, "Max"=1.0, "ScaleFac"=1.0, "ScaleOff"=0.0}, {"18F141F3", "Frame"="BMS05Error\ndatabase", "NameShort"="BMS05SOCTooLowWarn", "StartBit"=16, "NumBits"=1, "Min"=0.0, "Max"=1.0, "ScaleFac"=1.0, "ScaleOff"=0.0}, {"18F141F3", "Frame"="BMS05Error\ndatabase", "NameShort"="BMS05TempAbove75Warn", "StartBit"=22, "NumBits"=1, "Min"=0.0, "Max"=1.0, "ScaleFac"=1.0, "ScaleOff"=0.0}, {"18F141F3", "Frame"="BMS05Error\ndatabase", "NameShort"="BMS05TempAbove75WarnBoxNum", "StartBit"=27, "NumBits"=5, "Min"=0.0, "Max"=1.0, "ScaleFac"=1.0, "ScaleOff"=0.0}, {"18F141F3", "Frame"="BMS05Error\ndatabase", "NameShort"="BMS05TempDiffAbove30Warn", "StartBit"=8, "NumBits"=1, "Min"=0.0, "Max"=1.0, "ScaleFac"=1.0, "ScaleOff"=0.0}, {"18F141F3", "Frame"="BMS05Error\ndatabase", "NameShort"="BMS05UndervoltWarn", "StartBit"=11, "NumBits"=1, "Min"=0.0, "Max"=1.0, "ScaleFac"=1.0, "ScaleOff"=0.0}, {"18F142F3", "Frame"="BMS06\ndatabase", "NameShort"="BMS06BattMinTempPoint1", "StartBit"=0, "NumBits"=8, "Min"=-40.0, "Max"=210.0, "ScaleFac"=1.0, "ScaleOff"=-40.0}, {"18F142F3", "Frame"="BMS06\ndatabase", "NameShort"="BMS06BattMinTempPoint1BoxNum", "StartBit"=8, "NumBits"=8, "Min"=0.0, "Max"=100.0, "ScaleFac"=1.0, "ScaleOff"=0.0}, {"18F142F3", "Frame"="BMS06\n
